vi "Scan Engine Local Chassis.vi"(8 "error in (no error)":errorcluster, 11 "Node Ptr":T1 format="%.0x") -> (0 "error out":errorcluster)   [LabVIEW 2017, in "Scan Engine Custom Device.lvlib"]
uses:
  Scan Engine Custom Device.lvlib
  <vilib>/NI Veristand/Custom Device API/Custom Device Item Ref.ctl
  <vilib>/NI VeriStand/Custom Device API/Custom Device API.lvlib
  Scripting/Scan Engine Scripting.lvlib
panel:
  in  "SHDocVw.IWebBrowser2":refnum<k7>(container)
  in  "# Slots":i32 min=0 max=32
  in  "Header":cluster{"Section Name":string}={"Section Name"="Local Chassis Settings"}
  in  "Name":string
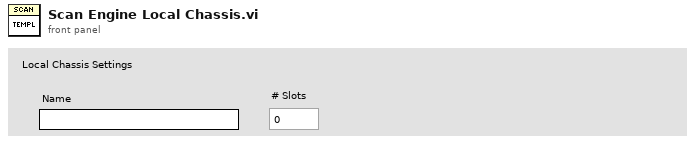
[diagram p1: front panel]
types:
  T1 = typedef "Custom Device API.lvlib/Custom Device Item Ref.ctl" = u64
  T2 = typedef "Custom Device API.lvlib/Custom Device Commands.ctl" = enum16{"Default", "Item renamed", "Shutdown", "Dynamic button pressed"}
  T3 = typedef "Custom Device API.lvlib/Custom Device Item Info.ctl" = cluster{"Name":string, "Is Channel":bool, "GUID":string, "Is Waveform":bool}
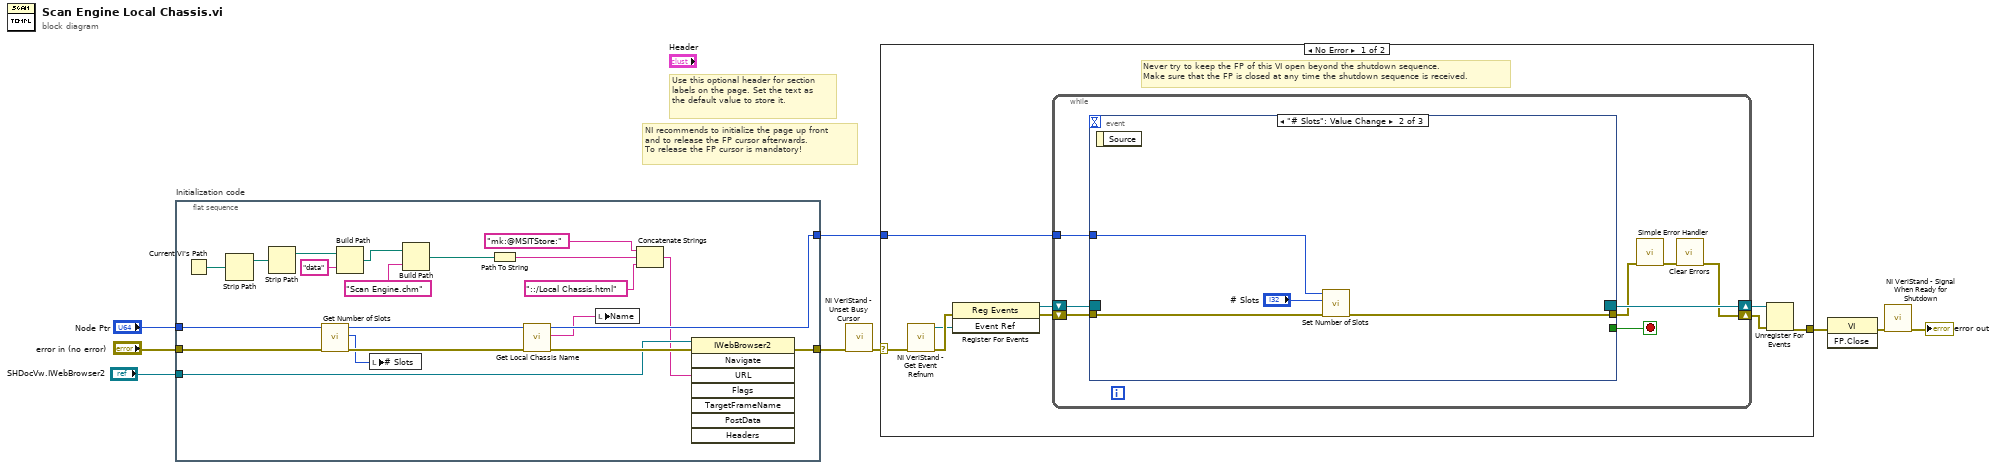
[diagram p0: block diagram]
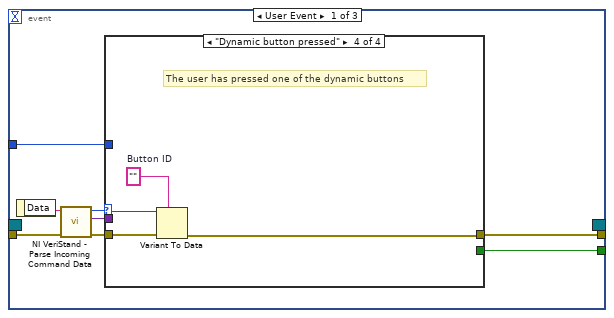
[diagram p2: hidden frame]
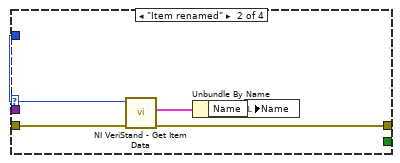
[diagram p4: hidden frame]
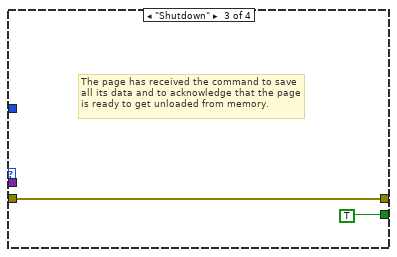
[diagram p5: hidden frame]
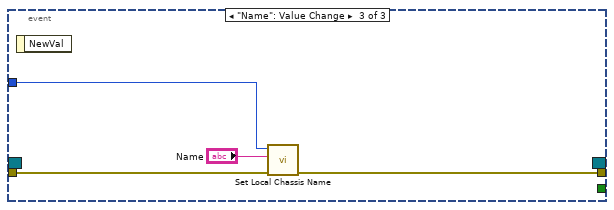
[diagram p6: hidden frame]
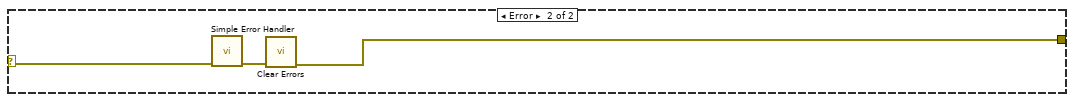
[diagram p7: hidden frame]
diagram:
  # "Use this optional header for section labels on the page. Set the text as the default value to store it."
  # "NI recommends to initialize the page up front\nand to release the FP cursor afterwards.\nTo release the FP cursor is mandatory!"
  n1 = flat-sequence "Initialization code" {
    tunnel: "error in (no error)" -> [w13]
    tunnel: "Node Ptr" -> [w14]
    tunnel: [w17] -> w5
    tunnel: [w30] -> w2
    tunnel: "SHDocVw.IWebBrowser2" -> [w16]
    frame #0 {
      n2 = Current VI's Path() -> (path=w27:path)
      n3 = Strip Path(path=w27) -> (stripped path=w26:path)  [unwired: 1 out]
      n4 = Strip Path(path=w26) -> (stripped path=w21:path)  [unwired: 1 out]
      n5 = call "Get Number of Slots.vi"("error in"=w13, "chassis ref in"=w14) -> ("error out"=w11:errorcluster, "number of slots"=w10:i32, "chassis ref out"=w12:T1)  [unwired: 7 in]
      n6 = Build Path(base path=w21, name or relative path="data") -> (appended path=w20:path)
      n7 = local write "# Slots"(w10) -> ()
      n8 = Build Path(base path=w20, name or relative path="Scan Engine.chm") -> (appended path=w23:path)
      n9 = Path To String(path=w23) -> (string=w24:string)
      n10 = call "Get Local Chassis Name.vi"("error in"=w11, "chassis ref in"=w12) -> ("error out"=w18:errorcluster, "name"=w29:string, "chassis ref out"=w30:T1)  [unwired: 7 in]
      n11 = local write "Name"(w29) -> ()
      n12 = Concatenate Strings("mk:@MSITStore:" ("string"), w24, "::/Local Chassis.html" ("name or relative path")) -> (w15:string)
      n13 = invoke class="IWebBrowser2" method="Navigate"(reference=w16, error in=w18, "URL"=w15) -> (error out=w17:errorcluster)  [unwired: 5 in, 7 out]
    }
  }
  n14 = call <vilib>:"NI VeriStand - Unset Busy Cursor.vi"("error in (no error)"=w5) -> ("error out"=w4:errorcluster)  [unwired: 10 out]
  n15 = case shown="No Error" w4 {
    selector: w4 -> [w31 w78]
    tunnel: [w36 w76] -> w9
    tunnel: w2 -> [w32 _]
    frame No Error {
      # "Never try to keep the FP of this VI open beyond the shutdown sequence.\nMake sure that the FP is closed at any time the shutdown sequence is received."
      n16 = call <vilib>:"NI VeriStand - Get Event Refnum.vi"("error in (no error)"=w31) -> ("error out"=w39:errorcluster, "Event Ref"=w35:refnum<user-event>)  [unwired: 9 out]
      n17 = register-events(error in=w39, w35) -> (reference out=w33:refnum<event-registration>, error out=w34:errorcluster)  [unwired: 1 in]
      n18 = while {
        tunnel: w32 -> [w43]
        shift-right: [w40] -> w37
        shift-left: w34 -> [w46]
        shift-right: [w47] -> w38
        shift-left: w33 -> [w45]
        stop <- w44 stop-if-true
        n19 = event shown="[1] \"# Slots\": Value Change" {
          selector: w45 -> [_ _ _]
          dyn-events: [_ _ _] -> w47
          timeout: _ -> [_ _ _]
          tunnel: w46 -> [w55 w71 w75]
          tunnel: [w51 _ _] -> w44
          tunnel: [w50 w70 w74] -> w42
          tunnel: w43 -> [w49 w69 w73]
          event User Event {
            n20 = event-data() -> ("Data"=w54:string)  [unwired: 1 out]
            n21 = call <vilib>:"NI VeriStand - Parse Incoming Command Data.vi"("error in (no error)"=w55, "Incoming data"=w54) -> ("error out"=w53:errorcluster, "Outgoing data"=w48:variant, "Action"=w52:T2)  [unwired: 7 out]
            n22 = case shown="\"Dynamic button pressed\"" w52 {
              tunnel: w53 -> [w56 w61 w62 w67]
              tunnel: [_ _ TRUE _] -> w51
              tunnel: [w56 w58 w62 w64] -> w50
              tunnel: w49 -> [_ w60 _ _]
              tunnel: w48 -> [_ _ _ w66]
              frame "Default", Default {
              }
              frame "Item renamed" {
                n23 = call <vilib>:"NI VeriStand - Get Item Data.vi"("error in (no error)"=w61, "Item Ref in"=w60) -> ("error out"=w58:errorcluster, "Item Info"=w59:T3)  [unwired: 8 out]
                n24 = Unbundle By Name(w59) -> ("Name"=w57:string)
                n25 = local write "Name"(w57) -> ()
              }
              frame "Shutdown" {
                # "The page has received the command to save all its data and to acknowledge that the page is ready to get unloaded from memory."
              }
              frame "Dynamic button pressed" {
                w65 = ""  # Button ID
                # "The user has pressed one of the dynamic buttons"
                n26 = Variant To Data(error in=w67, type=w65, Variant=w66) -> (error out=w64:errorcluster)  [unwired: 1 out]
              }
            }
          }
          event "# Slots": Value Change {
            n27 = event-data() -> ()  [unwired: 2 out]
            n28 = call "Set Number of Slots.vi"("error in"=w71, "number of slots"="# Slots", "chassis ref in"=w69) -> ("error out"=w70:errorcluster)  [unwired: 7 in, 1 out]
          }
          event "Name": Value Change {
            n29 = event-data() -> ()  [unwired: 2 out]
            n30 = call "Set Local Chassis Name.vi"("error in"=w75, "name"="Name", "chassis ref in"=w73) -> ("error out"=w74:errorcluster)  [unwired: 8 in]
          }
        }
        n31 = call <vilib>:"Simple Error Handler.vi"("error in (no error)"=w42) -> ("error out"=w41:errorcluster)  [unwired: 1 in, 7 out]
        n32 = call <vilib>:"Clear Errors.vi"("error in (no error)"=w41) -> ("error out"=w40:errorcluster)  [unwired: 1 in, 5 out]
      }
      n33 = Unregister For Events(event registration refnum=w38, error in=w37) -> (error out=w36:errorcluster)
    }
    frame Error {
      n34 = call <vilib>:"Simple Error Handler.vi"("error in (no error)"=w78) -> ("error out"=w77:errorcluster)  [unwired: 1 in, 7 out]
      n35 = call <vilib>:"Clear Errors.vi"("error in (no error)"=w77) -> ("error out"=w76:errorcluster)  [unwired: 1 in, 5 out]
    }
  }
  n36 = invoke class="VI" method="FP.Close"(error in=w9) -> (error out=w8:errorcluster)  [unwired: 2 in, 2 out]
  n37 = call <vilib>:"NI VeriStand - Signal When Ready for Shutdown.vi"("error in (no error)"=w8) -> ("error out"=→"error out":errorcluster)  [unwired: 10 out]
